vi "Store Session Reservation.vi"(8 "error in":errorcluster, 10 "session reservation":refnum<class "Session Reservation.lvclass">, 11 "measurement context in":refnum<class "MeasurementContext.lvclass">) -> (0 "error out":errorcluster, 3 "measurement context out":refnum<class "MeasurementContext.lvclass">)   [LabVIEW 2020, in "MeasurementLink Measurement Server.lvlib" / "MeasurementContext.lvclass"]
uses:
  MeasurementContext.lvclass
  MeasurementContext.lvclass/MeasurementContext.ctl
  MeasurementLink Session Management/Session Reservation/Session Reservation.lvclass
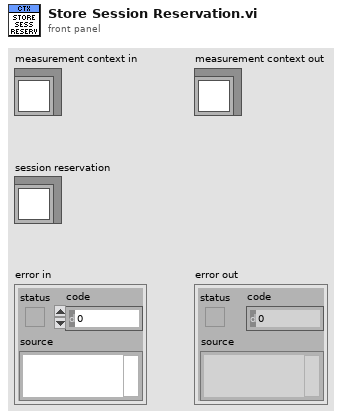
[diagram p1: front panel]
types:
  T1 = typedef "MeasurementLink Measurement Server.lvlib/MeasurementContext.lvclass/Data.ctl" = cluster{"PinMapContext":T2, "gRPCServerId":T3, "IMeasurementService":refnum<class "IMeasurementService.lvclass">, "MeasurementPluginService":refnum<class "MeasurementPluginService.lvclass">, "Session Reservations":refnum<class "Session Reservation.lvclass">[]}
  T2 = typedef "MeasurementLink Measurement Server.lvlib/PinMapContext.ctl" = cluster{"pin_map_id":string, "sites":i32[]}
  T3 = typedef "grpc-lvsupport-release.lvlib/grpcId.ctl" = u64
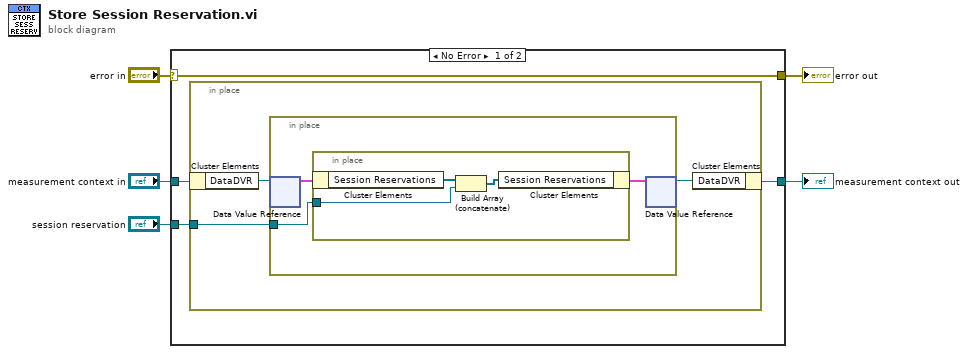
[diagram p0: block diagram]
diagram:
  n1 = case shown="No Error" "error in" {
    selector: "error in" -> [w8 w20]
    tunnel: [w8 w20] -> w4
    tunnel: [w7 w19] -> w2
    tunnel: "measurement context in" -> [w9 w19]
    tunnel: "session reservation" -> [w6 _]
    frame No Error {
      n2 = in-place {
        in-place-border: w6 -> [w10]
        n3 = in-place-cluster #1(w9) -> ("DataDVR"=w12:refnum<data-value>)
        n4 = in-place {
          in-place-border: w10 -> [w13]
          n5 = in-place-dvr #2(w12) -> (w15:T1)  [unwired: 1 out]
          n6 = in-place {
            in-place-border: w13 -> [w16]
            n7 = in-place-cluster #3(w15) -> ("Session Reservations"=w18:refnum<class "Session Reservation.lvclass">[])
            n8 = Build Array (concatenate)(w18, w16) -> (w17:refnum<class "Session Reservation.lvclass">[])
            n9 = in-place-cluster #3("Session Reservations"=w17) -> (w14:T1)
          }
          n10 = in-place-dvr #2(w14) -> (w11:refnum<data-value>)  [unwired: 1 out]
        }
        n11 = in-place-cluster #1("DataDVR"=w11) -> (w7:refnum<class "MeasurementContext.lvclass">)
      }
    }
    frame Error {
    }
  }
  "error out" <- w4
  "measurement context out" <- w2
